vi "dummy_report_read.vi"() -> ()   [LabVIEW 2014]
uses:
  control/FGV Serial Tasks.ctl
panel:
  out "return count":u32
  out "read buffer":string
  in  "String":string="H"
  in  "VISA resource name":refnum<visa-resource-name>="COM3"
  # "0130 3152 5233 43\n00 0000 0000 0000 0000 0000 0000 0262 0000 0000 008A 21D8 0000 0000 568F CF00 \n     0000 0000 0000 0000 0000 0000 0262 0000 0000 0076 21D9 0000 0000 5690 8B35 42\n04"
  # "0130 3152 5233 4300 0000 0000 0000 0000 0000 0000 0262 0000 0000 008A 21D8 0000 0000 568F CF00 0000 0000 0000 0000 0000 0000 0262 0000 0000 0076 21D9 0000 0000 5690 8B35 4204"
  # "0130 3152 5233 4300 0000 0000 0000 0000 0000 0000 0262 0000 0000 008A 21D8 0000 0000 568F CF00 0000 0000 0000 0000 0000 0000 0262 0000 0000 0076 21D9 0000 0000 5690 8B35 4204"
  # "0130 3152 5233 4300 0000 0000 0000 0000 0000 0000 0262 0000 0000 008A 21D8 0000 0000 568F CF00 0000 0000 0000 0000 0000 0000 0262 0000 0000 0076 21D9 0000 0000 5690 8B35 4204"
  # "0130 3152 5233 4300 0000 0000 0000 0000 0000 0000 0262 0000 0000 0079 21F9 0000 0000 56AC EC00 0000 0000 0000 0000 0000 0000 0262 0000 0000 0079 21FA 0000 0000 56AD A446 4604"
  # "0130 3152 5233 4300 0000 0000 0000 0000 0000 0000 0262 0000 0000 0079 21FC 0000 0000 56AE F400 0000 0000 0000 0000 0000 0000 0262 0000 0000 0076 21FD 0000 0000 56AF B832 3204"
  # "0130 3152 5233 4300 0000 0000 0000 0000 0000 0000 0262 0000 0000 007C 2260 0000 0000 56F3 5600 0000 0000 0000 0000 0000 0000 0262 0000 0000 0076 2261 0000 0000 56F3 CD45 4604"
  # "0130 3152 5233 4300 0000 0000 0000 0000 0000 0000 0262 0000 0000 007C 2260 0000 0000 56F3 5600 0000 0000 0000 0000 0000 0000 0262 0000 0000 0076 2261 0000 0000 56F3 CD45 4604"
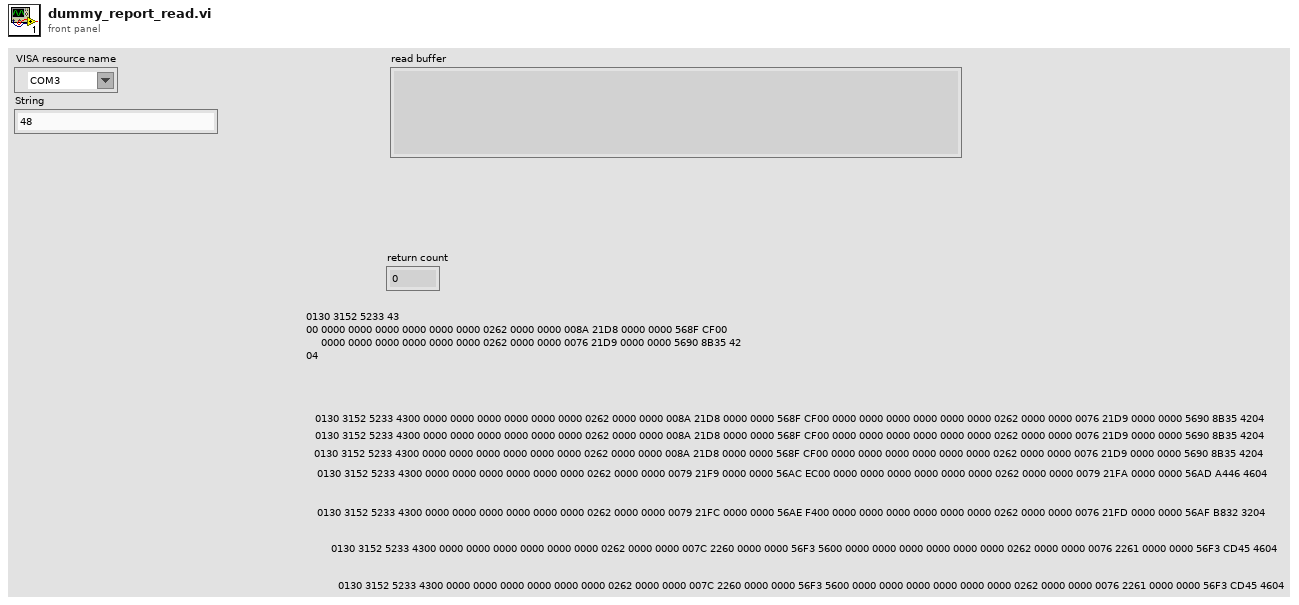
[diagram p1: front panel]
types:
  T1 = typedef "FGV Serial Tasks.ctl" = enum16{"Open", "Read", "Write", "Close", "Flush"}
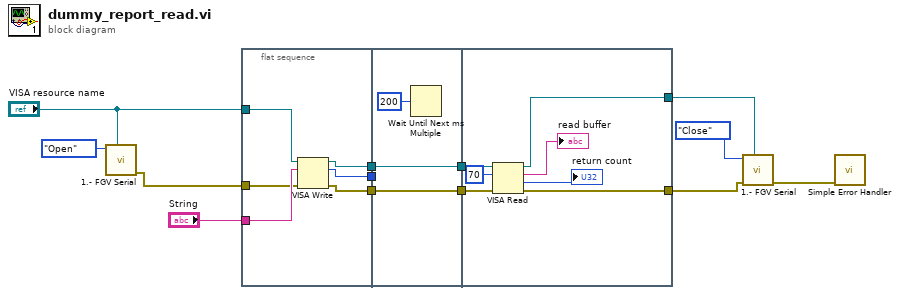
[diagram p0: block diagram]
diagram:
  n1 = call "1.- FGV Serial.vi"("VISA resource name"="VISA resource name", "Task"=FGV_Serial_Tasks."Open") -> ("error out"=w10:errorcluster)  [unwired: 7 in, 2 out]
  n2 = flat-sequence {
    tunnel: "VISA resource name" -> [w19]
    tunnel: "String" -> [w18]
    tunnel: w10 -> [w17]
    tunnel: [w16] -> w8
    tunnel: [w15] -> w7
    tunnel: [w14] -> w5
    tunnel: [w21] -> w9
    tunnel: w8 -> [w21]
    tunnel: w7 -> [_]
    tunnel: [w20] -> w6
    tunnel: w5 -> [w20]
    tunnel: w9 -> [w29]
    tunnel: w6 -> [w28]
    tunnel: [w25] -> w3
    tunnel: [w24] -> w2
    frame #0 {
      n3 = VISA Write(VISA resource name=w19, write buffer=w18, error in (no error)=w17) -> (VISA resource name out=w16:refnum<visa-resource-name>, return count=w15:u32, error out=w14:errorcluster)
    }
    frame #1 {
      n4 = Wait Until Next ms Multiple(millisecond multiple=u32 200) -> ()  [unwired: 1 out]
    }
    frame #2 {
      n5 = VISA Read(VISA resource name=w29, byte count=u32 70, error in (no error)=w28) -> (VISA resource name out=w24:refnum<visa-resource-name>, read buffer=→"read buffer":string, return count=→"return count":u32, error out=w25:errorcluster)
    }
  }
  n6 = call "1.- FGV Serial.vi"("VISA resource name"=w2, "error in (no error)"=w3, "Task"=FGV_Serial_Tasks."Close") -> ("error out"=w1:errorcluster)  [unwired: 6 in, 2 out]
  n7 = call <vilib>:"Simple Error Handler.vi"("error in (no error)"=w1) -> ()  [unwired: 4 in, 5 out]
